vi "_Publish Group.vi"(8 "error in (no error)":errorcluster, 10 "Publish Group Data":T1, 11 "Loop Data In":T4) -> (0 "error out":errorcluster, 3 "Loop Data":T4)   [LabVIEW 2020, in "Vecto.lvlib" / "RemoteDataService.lvclass"]
uses:
  RemoteDataService.lvclass
  Loop Data.ctl
  SequenceCountService/SequenceCountService.lvclass
  ChannelService/ChannelService.lvclass
  Published Group.ctl
  Packet.ctl
  lv-protoc/LV-Proto/Message/Message.lvclass
  Group Data Type.ctl
  Subscription.ctl
  Subscription Info.ctl
  SubscribedDataHandler/SubscribedDataHandler.lvclass
  VectoConfig/Telemetry Config.ctl
  VectoConfig/Telemetry Routing.ctl
  VectoConfig/Endpoint.ctl
  Publish Group Data.ctl
  4fb0fbe4-9380-471d-b238-2622956b2100.vi
  a382f260-bea0-4ad7-9574-7ab04d3346eb.vi
  9f550317-846c-4a38-96e8-0692b9bc9e9f.vi
  ae571fe3-6f9a-499d-bd4d-f6e66c0965c2.vi
  27333bca-8783-4ec9-bc13-b6d6669e9723.vi
  <vilib>/Utility/High Resolution Relative Seconds.vi
  RemoteDataService.lvclass/RemoteDataService.ctl
  VectoConfig/VectoConfig.lvlib
panel:
  out "Chart":T3(graph)
  out "Enqueue":dbl format="%#_6f"
  out "Build Message":dbl format="%#_6f"
  out "Map Lookup":dbl format="%#_6f"
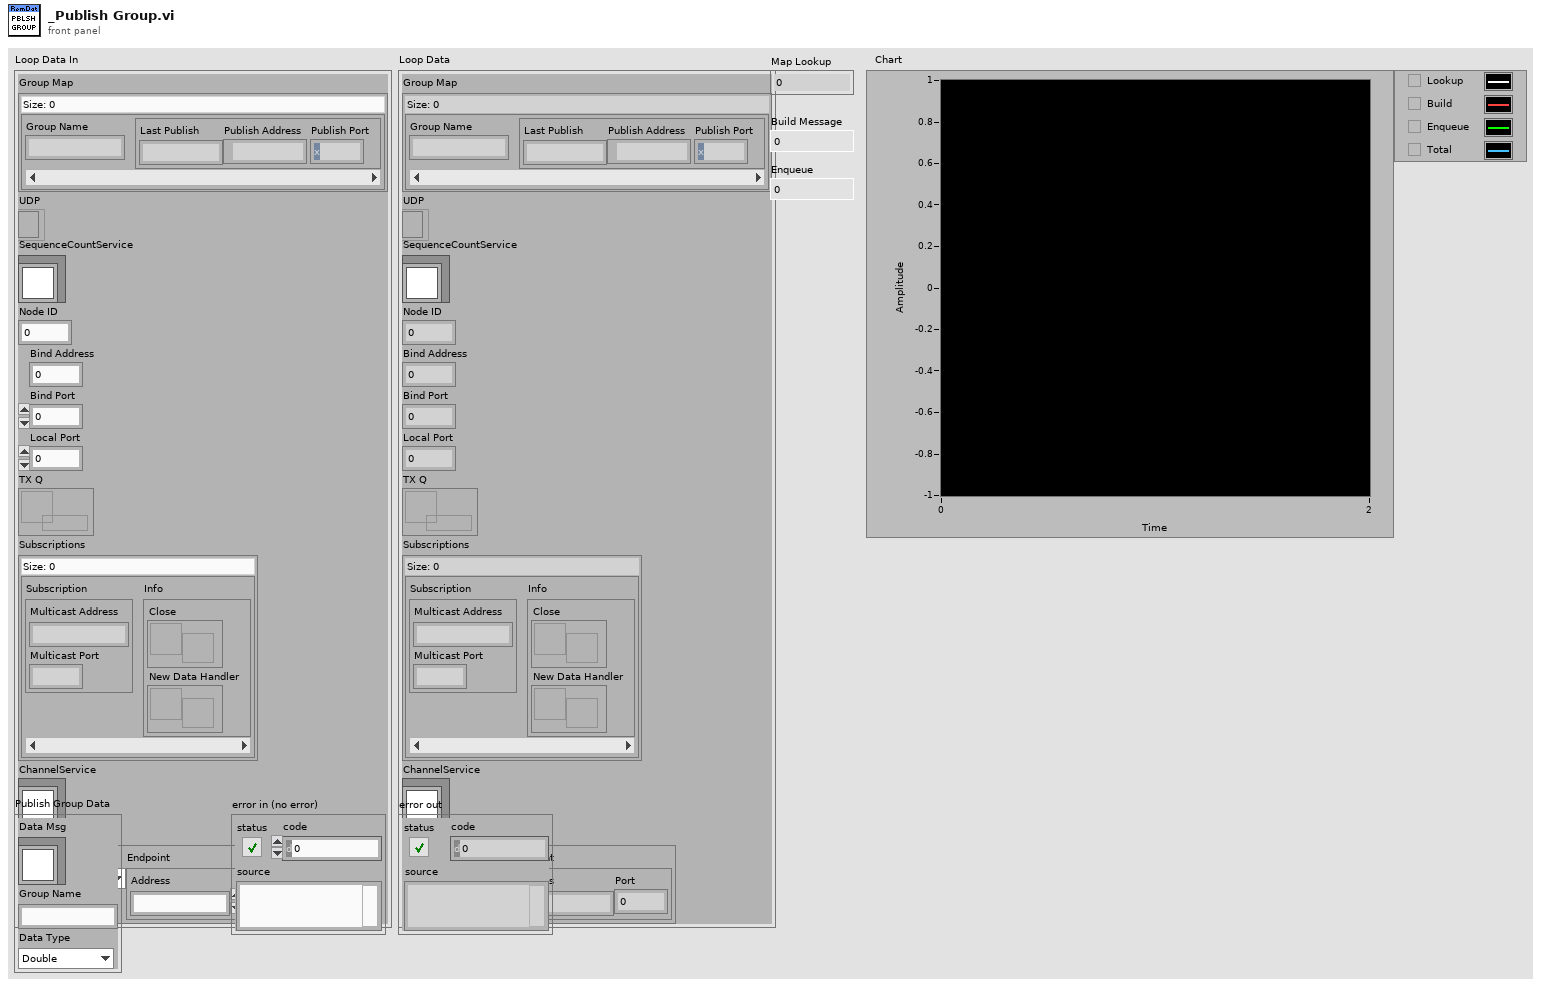
[diagram p1: front panel]
types:
  T1 = typedef "Vecto.lvlib/RemoteDataService.lvclass/Publish Group Data.ctl" = cluster{"Data Msg":refnum<class "Message.lvclass">, "Group Name":string, "Data Type":T2}
  T2 = typedef "VectoConfig.lvlib/Group Data Type.ctl" = enum16{"Double", "String", "Bool"}
  T3 = cluster{"Delta":dbl, "Delta":dbl, "Delta":dbl, "Delta":dbl}
  T4 = typedef "Vecto.lvlib/RemoteDataService.lvclass/Loop Data.ctl" = cluster{"Group Map":map{string, T5}, "UDP":refnum<k16>, "SequenceCountService":refnum<class "SequenceCountService.lvclass">, "Node ID":u32, "Bind Address":u32, "Bind Port":u16, "Local Port":u16, "TX Q":refnum<queue>, "Subscriptions":map{T6, T7}, "ChannelService":refnum<class "ChannelService.lvclass">, "Telemetry Config":T8}
  T5 = typedef "Vecto.lvlib/RemoteDataService.lvclass/Published Group.ctl" = cluster{"Last Publish":dbl, "Publish Address":u32, "Publish Port":u16}
  T6 = typedef "Vecto.lvlib/RemoteDataService.lvclass/Subscription.ctl" = cluster{"Multicast Address":string, "Multicast Port":u16}
  T7 = typedef "Vecto.lvlib/RemoteDataService.lvclass/Subscription Info.ctl" = cluster{"Close":refnum<user-event>, "New Data Handler":refnum<user-event>}
  T8 = typedef "VectoConfig.lvlib/Telemetry Config.ctl" = cluster{"Routing":T9, "Endpoint":T10}
  T9 = typedef "VectoConfig.lvlib/Telemetry Routing.ctl" = enum16{"Multicast", "Unicast"}
  T10 = typedef "VectoConfig.lvlib/Endpoint.ctl" = cluster{"Address":string, "Port":u16}
  T11 = typedef "Vecto.lvlib/RemoteDataService.lvclass/Packet.ctl" = cluster{"UDP":refnum<k16>, "IP":u32, "Port":u16, "Message":refnum<class "Message.lvclass">, "Data Type":T2}
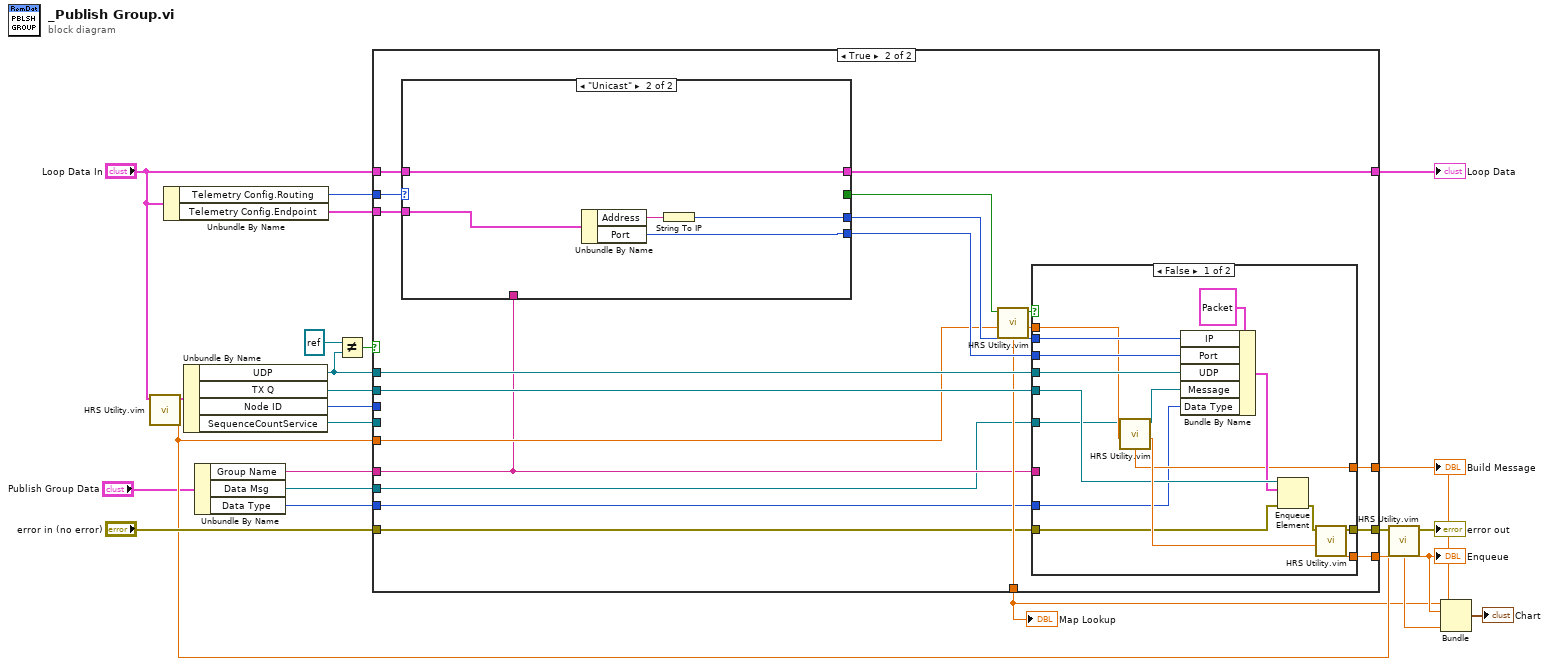
[diagram p0: block diagram]
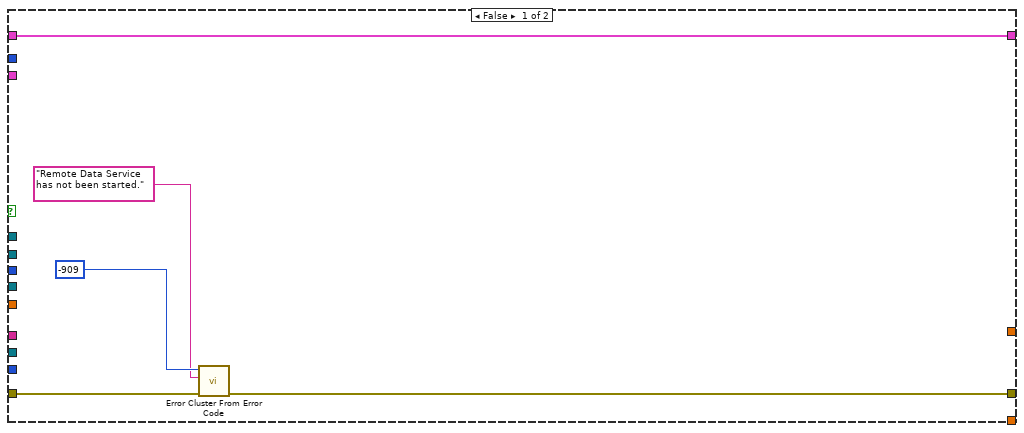
[diagram p2: hidden frame]
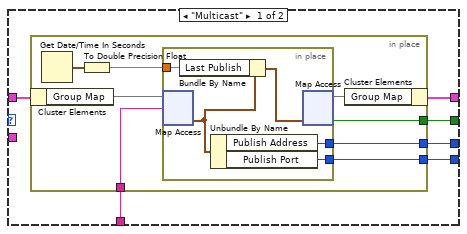
[diagram p3: hidden frame]
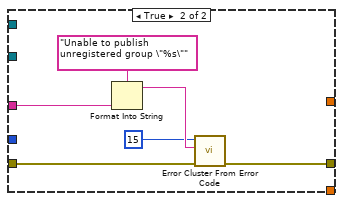
[diagram p4: hidden frame]
diagram:
  n1 = call "HRS Utility.vim"("In"="Loop Data In") -> ("Out"=w16:T4, "HRS"=w10:dbl)  [unwired: 6 in, 1 out]
  n2 = Unbundle By Name("Loop Data In") -> ("Telemetry Config.Routing"=w2:T9, "Telemetry Config.Endpoint"=w1:T10)
  n3 = Unbundle By Name(w16) -> ("UDP"=w20:refnum<k16>, "TX Q"=w19:refnum<queue>, "Node ID"=w18:u32, "SequenceCountService"=w17:refnum<class "SequenceCountService.lvclass">)
  n4 = Unbundle By Name("Publish Group Data") -> ("Group Name"=w6:string, "Data Msg"=w5:refnum<class "Message.lvclass">, "Data Type"=w4:T2)
  n5 = Not Equal?(x=refnum<k16> refnum, y=w20) -> (x != y?=w21:bool)
  n6 = case shown="True" w21 {
    tunnel: "Loop Data In" -> [w29 w49]
    tunnel: "error in (no error)" -> [w28 w33]
    tunnel: w5 -> [_ w34]
    tunnel: [w29 w48] -> w24
    tunnel: [w27 w47] -> w23
    tunnel: w20 -> [_ w46]
    tunnel: w19 -> [_ w45]
    tunnel: w18 -> [_ _]
    tunnel: w17 -> [_ _]
    tunnel: [_ w44] -> w12
    tunnel: [_ w43] -> w15
    tunnel: w10 -> [_ w38]
    tunnel: [_ w36] -> w9
    tunnel: w6 -> [_ w35]
    tunnel: w4 -> [_ w32]
    tunnel: w2 -> [_ w31]
    tunnel: w1 -> [_ w30]
    frame False {
      n7 = call <vilib>:"Error Cluster From Error Code.vi"("error in (no error)"=w28, "error message (\"\")"="Remote Data Service has not been started.", "error code (0)"=-909) -> ("error out"=w27:errorcluster)  [unwired: 6 in]
    }
    frame True {
      n8 = case shown="\"Unicast\"" w31 {
        tunnel: w49 -> [w55 w73]
        tunnel: [w54 w73] -> w48
        tunnel: [w53 w69] -> w42
        tunnel: [w52 w70] -> w41
        tunnel: [w51 _] -> w40
        tunnel: w35 -> [w50 _]
        tunnel: w30 -> [_ w72]
        frame "Multicast" {
          n9 = in-place {
            in-place-border: [w61] -> w53
            in-place-border: [w60] -> w52
            in-place-border: w50 -> [w58]
            in-place-border: [w56] -> w51
            n10 = in-place-cluster #1(w55) -> ("Group Map"=w59:map{string, T5})
            n11 = Get Date/Time In Seconds() -> (seconds since 1Jan1904=w63:timestamp)
            n12 = To Double Precision Float(number=w63) -> (double precision float=w62:dbl)
            n13 = in-place {
              in-place-border: w62 -> [w68]
              in-place-border: [w67] -> w61
              in-place-border: [w66] -> w60
              n14 = in-place-map #2(w59, w58) -> (w65:T5)  [unwired: 1 in, 1 out]
              n15 = Bundle By Name(cluster=w65, "Last Publish"=w68) -> (w64:T5)
              n16 = Unbundle By Name(w65) -> ("Publish Address"=w66:u32, "Publish Port"=w67:u16)
              n17 = in-place-map #2(w64) -> (w57:map{string, T5}, w56:bool)  [unwired: 1 in, 1 out]
            }
            n18 = in-place-cluster #1("Group Map"=w57) -> (w54:T4)
          }
        }
        frame "Unicast" {
          n19 = Unbundle By Name(w72) -> ("Address"=w71:string, "Port"=w69:u16)
          n20 = String To IP(1:w71) -> (0:w70:u32)
        }
      }
      n21 = call "HRS Utility.vim"("In"=w40, "Prev"=w38) -> ("Out"=w39:bool, "HRS"=w37:dbl, "Delta"=w36:dbl)  [unwired: 5 in]
      n22 = case shown="False" w39 {
        tunnel: w33 -> [w76 w92]
        tunnel: [w89 w91] -> w47
        tunnel: w46 -> [w88 _]
        tunnel: w45 -> [w81 _]
        tunnel: [w79 _] -> w44
        tunnel: [w87 _] -> w43
        tunnel: w34 -> [w75 _]
        tunnel: w42 -> [w83 _]
        tunnel: w41 -> [w82 _]
        tunnel: w37 -> [w78 _]
        tunnel: w35 -> [_ w90]
        tunnel: w32 -> [w74 _]
        frame False {
          n23 = call "HRS Utility.vim"("In"=w75, "Prev"=w78) -> ("Out"=w77:refnum<class "Message.lvclass">, "HRS"=w84:dbl, "Delta"=w79:dbl)  [unwired: 5 in]
          n24 = Bundle By Name(cluster=T11 {"UDP"=refnum, "IP"=0, "Port"=0, "Message"=refnum, "Data Type"=enum."Double"} ("Packet"), "IP"=w82, "Port"=w83, "UDP"=w88, "Message"=w77, "Data Type"=w74) -> (w80:T11)
          n25 = Enqueue Element(queue=w81, element=w80, error in (no error)=w76) -> (error out=w85:errorcluster)  [unwired: 1 in, 2 out]
          n26 = call "HRS Utility.vim"("In"=w85, "Prev"=w84) -> ("Out"=w89:errorcluster, "Delta"=w87:dbl)  [unwired: 5 in, 1 out]
        }
        frame True {
          n27 = Format Into String(format string="Unable to publish unregistered group \"%s\"", w90) -> (resulting string=w95:string)  [unwired: 2 in, 1 out]
          n28 = call <vilib>:"Error Cluster From Error Code.vi"("error in (no error)"=w92, "error message (\"\")"=w95, "error code (0)"=15) -> ("error out"=w91:errorcluster)  [unwired: 6 in]
        }
      }
    }
  }
  "Loop Data" <- w24
  "Map Lookup" <- w9
  "Build Message" <- w12
  "Enqueue" <- w15
  n29 = call "HRS Utility.vim"("In"=w23, "Prev"=w10) -> ("Out"=→"error out":errorcluster, "Delta"=w13:dbl)  [unwired: 5 in, 1 out]
  n30 = Bundle("Delta"=w9, "Delta"=w15, "Delta"=w12, "Delta"=w13) -> (→"Chart":T3)  [unwired: 1 in]
